vi "Get MD5 for File.vi"(8 "error in":errorcluster, 11 "Path":path) -> (0 "error out":errorcluster, 1 "MD5":string)   [LabVIEW 2020]
uses:
  NationalInstruments.VeriStand.Internal
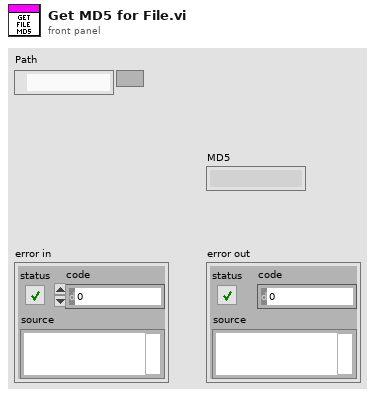
[diagram p1: front panel]
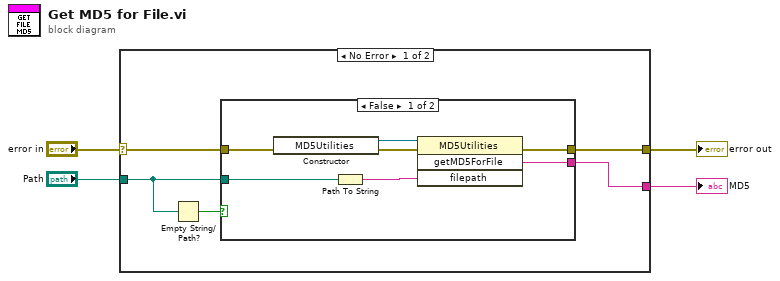
[diagram p0: block diagram]
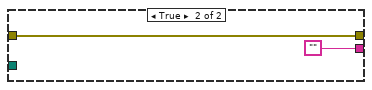
[diagram p2: hidden frame]
diagram:
  n1 = case shown="No Error" "error in" {
    selector: "error in" -> [w9 w19]
    tunnel: "Path" -> [w7 _]
    tunnel: [w6 _] -> w1
    tunnel: [w5 w19] -> w2
    frame No Error {
      n2 = Empty String/Path?(string/path=w7) -> (empty?=w8:bool)
      n3 = case shown="False" w8 {
        tunnel: w9 -> [w16 w18]
        tunnel: w7 -> [w10 _]
        tunnel: [w12 w18] -> w5
        tunnel: [w13 ""] -> w6
        frame False {
          n4 = constructor class="MD5Utilities"(error in=w16) -> (reference out=w15:refnum<k24>, error out=w14:errorcluster)  [unwired: 2 in, 1 out]
          n5 = Path To String(path=w10) -> (string=w11:string)
          n6 = invoke class="MD5Utilities" method="getMD5ForFile"(reference=w15, error in=w14, "filepath"=w11) -> (error out=w12:errorcluster, "getMD5ForFile"=w13:string)  [unwired: 1 in, 2 out]
        }
        frame True {
        }
      }
    }
    frame Error {
    }
  }
  "error out" <- w2
  "MD5" <- w1
